vi "Attenuator Scale Graphs.vi"(8 "Attenuator Test Parameters":T1={"Stimulus"={"ATT Stimulus"={"Normalize"=TRUE, "Value (dB)"=0.0}, "VNA Stimulus"={"Use Instrument Settings"=FALSE, "Blank Frequencies"=FALSE, "Sweep Type"=enum."Linear", "Sweep"={"Fstart"=500.0, "Fstop"=1500.0, "Units"=enum."MHz", "Points"=201}, "Power (dBm)"=999.0, "IFBW (Hz)"=-1.0, "Sweep Time (s)"=-1.0, "Calibration"={"State"=FALSE, "String"=""}}}, "Measurement"={"Step (dB)"=enum."0.25", "Start (dB)"=0.0, "Stop (dB)"=31.75}, "Limit"={"Maximum Error"=0.3}, "Normalization"={"Normalized?"=FALSE, "Normalization Values (dB)"=[]}} {"Stimulus"."VNA Stimulus"."Sweep Time (s)" format="%.3g"}, 10 "Attenuation Variance":refnum<vi>, 11 "Frequency":refnum<vi>) -> ()   [LabVIEW 2011]
uses:
  TypeDefs/Attenuator Test Parameters.ctl
  TypeDefs/Attenuator Stimulus Parameters.ctl
  TypeDefs/Attenuator ATT Stimulus.ctl
  TypeDefs/Attenuator VNA Stimulus.ctl
  S Parameter/TypeDefs/SP Frequency Units.ctl
  TypeDefs/Attenuator VNA Calibration State.ctl
  TypeDefs/Attenuator Measurement Cluster.ctl
  TypeDefs/Attenuator Limit.ctl
  TypeDefs/Attenuator Calibration State.ctl
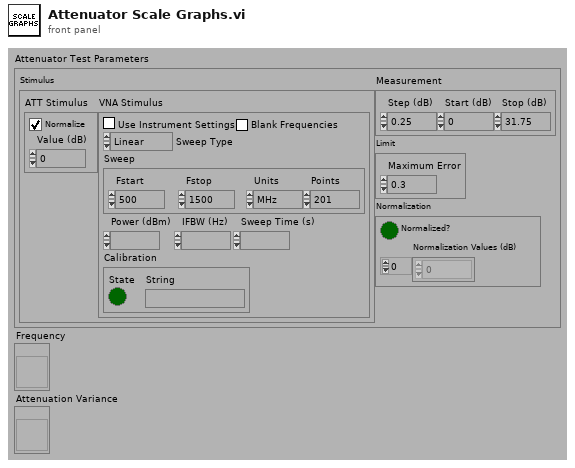
[diagram p1: front panel]
types:
  T1 = typedef "Attenuator Test Parameters.ctl" = cluster{"Stimulus":T2, "Measurement":T7, "Limit":T8, "Normalization":T9}
  T2 = typedef "Attenuator Stimulus Parameters.ctl" = cluster{"ATT Stimulus":T3, "VNA Stimulus":T4}
  T3 = typedef "Attenuator ATT Stimulus.ctl" = cluster{"Normalize":bool, "Value (dB)":dbl}
  T4 = typedef "Attenuator VNA Stimulus.ctl" = cluster{"Use Instrument Settings":bool, "Blank Frequencies":bool, "Sweep Type":enum32{"Linear", "Logarithmic", "List", "Power", "CW"}, "Sweep":cluster{"Fstart":dbl, "Fstop":dbl, "Units":T5, "Points":i32}, "Power (dBm)":dbl, "IFBW (Hz)":dbl, "Sweep Time (s)":dbl, "Calibration":T6}
  T5 = typedef "SP Frequency Units.ctl" = enum16{"Hz", "kHz", "MHz", "GHz", "Points"}
  T6 = typedef "Attenuator VNA Calibration State.ctl" = cluster{"State":bool, "String":string}
  T7 = typedef "Attenuator Measurement Cluster.ctl" = cluster{"Step (dB)":enum16{"0.25", "0.50", "1.00"}, "Start (dB)":dbl, "Stop (dB)":dbl}
  T8 = typedef "Attenuator Limit.ctl" = cluster{"Maximum Error":dbl}
  T9 = typedef "Attenuator Calibration State.ctl" = cluster{"Normalized?":bool, "Normalization Values (dB)":dbl[]}
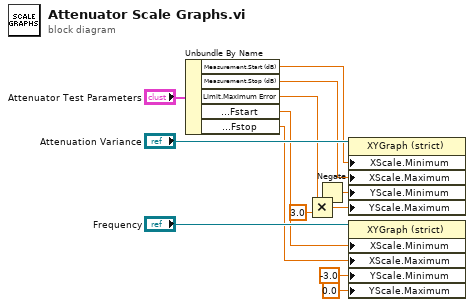
[diagram p0: block diagram]
diagram:
  n1 = Unbundle By Name("Attenuator Test Parameters") -> ("Measurement.Start (dB)"=w11:dbl, "Measurement.Stop (dB)"=w10:dbl, "Limit.Maximum Error"=w9:dbl, "Stimulus.VNA Stimulus.Sweep.Fstart"=w4:dbl, "Stimulus.VNA Stimulus.Sweep.Fstop"=w3:dbl)
  n2 = Multiply(x=w9, y=3.0) -> (x*y=w6:dbl)
  n3 = Negate(x=w6) -> (-x=w7:dbl)
  n4 = property class="XYGraph (strict)"(reference="Attenuation Variance", "XScale.Minimum"=w11, "XScale.Maximum"=w10, "YScale.Minimum"=w7, "YScale.Maximum"=w6) -> ()  [unwired: 1 in, 2 out]
  n5 = property class="XYGraph (strict)"(reference="Frequency", "XScale.Minimum"=w4, "XScale.Maximum"=w3, "YScale.Minimum"=-3.0 ("Y Scale.Range:Minimum"), "YScale.Maximum"=0.0 ("Y Scale.Range:Maximum")) -> ()  [unwired: 1 in, 2 out]
